vi "Read AppOutputData.vi"(8 "error in (no error)":errorcluster, 11 "AppPluginsBase in":refnum<class "AppPluginsBase.lvclass">) -> (0 "error out":errorcluster, 2 "AppOutputData":variant, 3 "AppPluginsBase out":refnum<class "AppPluginsBase.lvclass">)   [LabVIEW 2017, in "AppPlugins.lvlib" / "AppPluginsBase.lvclass"]
uses:
  AppPluginsBase.lvclass
  AppPluginsBase.lvclass/AppPluginsBase.ctl
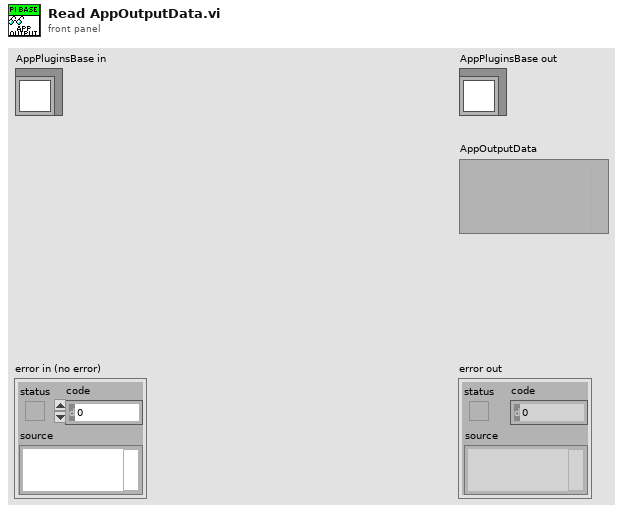
[diagram p1: front panel]
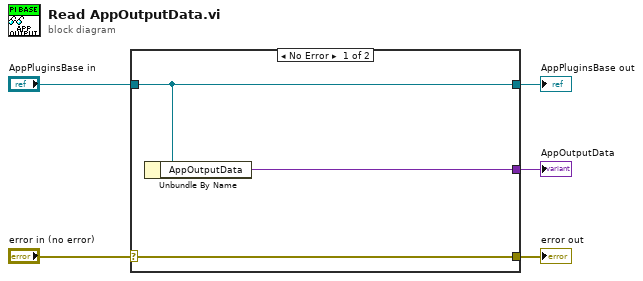
[diagram p0: block diagram]
diagram:
  n1 = case shown="No Error" "error in (no error)" {
    selector: "error in (no error)" -> [w8 w9]
    tunnel: [w8 w9] -> w4
    tunnel: [w7 w10] -> w2
    tunnel: "AppPluginsBase in" -> [w7 w10]
    tunnel: [w6 _] -> w1
    frame No Error {
      n2 = Unbundle By Name(w7) -> ("AppOutputData"=w6:variant)
    }
    frame Error {
    }
  }
  "error out" <- w4
  "AppPluginsBase out" <- w2
  "AppOutputData" <- w1
